vi "Append Image to Report (path).vi"(0 "report in":refnum<class "ooWriter.lvclass">, 1 "alignment (default)":T1, 2 "MS Office parameters":T2, 7 "path or URL of image":path, 9 "caption or alternative string":string, 11 "error in (no error)":errorcluster) -> (4 "report out":refnum<class "ooWriter.lvclass">, 8 "start out (Word)":i32, 10 "end out (Word)":i32, 15 "error out":errorcluster)   [LabVIEW 2009, in "ooWriter.lvclass"]
doc: "For an HTML report, the VI embeds a link to an image into the report. For a standard report, the VI appends the image from a file. You can wire either a path to the image or a string that contains the image URL to this polymorphic VI. The data type you wire to the <B>path or URL of image</B> input determines the polymorphic instance to use."
uses:
  ooWriter.lvclass
  <vilib>/Utility/NIReport.llb/HTML Report Image Alignment.ctl
  C:/Projets/LAVAG/OpenOfficeRGT/AODL/DLLs/AODL.dll
  ooWriter.lvclass/ooWriter.ctl
  <vilib>/Utility/NIReport.llb/NI_ReportGenerationCore.lvlib
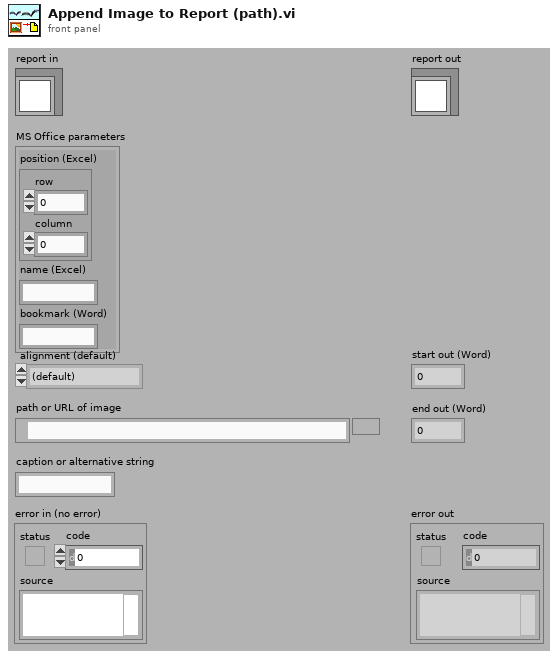
[diagram p1: front panel]
types:
  T1 = typedef "NI_ReportGenerationCore.lvlib/HTML Report Image Alignment.ctl" = enum16{"(default)", "LEFT", "RIGHT", "TOP", "TEXTTOP", "MIDDLE", "ABSMIDDLE", "BASELINE", "BOTTOM", "ABSBOTTOM"}
  T2 = cluster{"position (Excel)":cluster{"row":i32, "column":i32}, "name (Excel)":string, "bookmark (Word)":string}
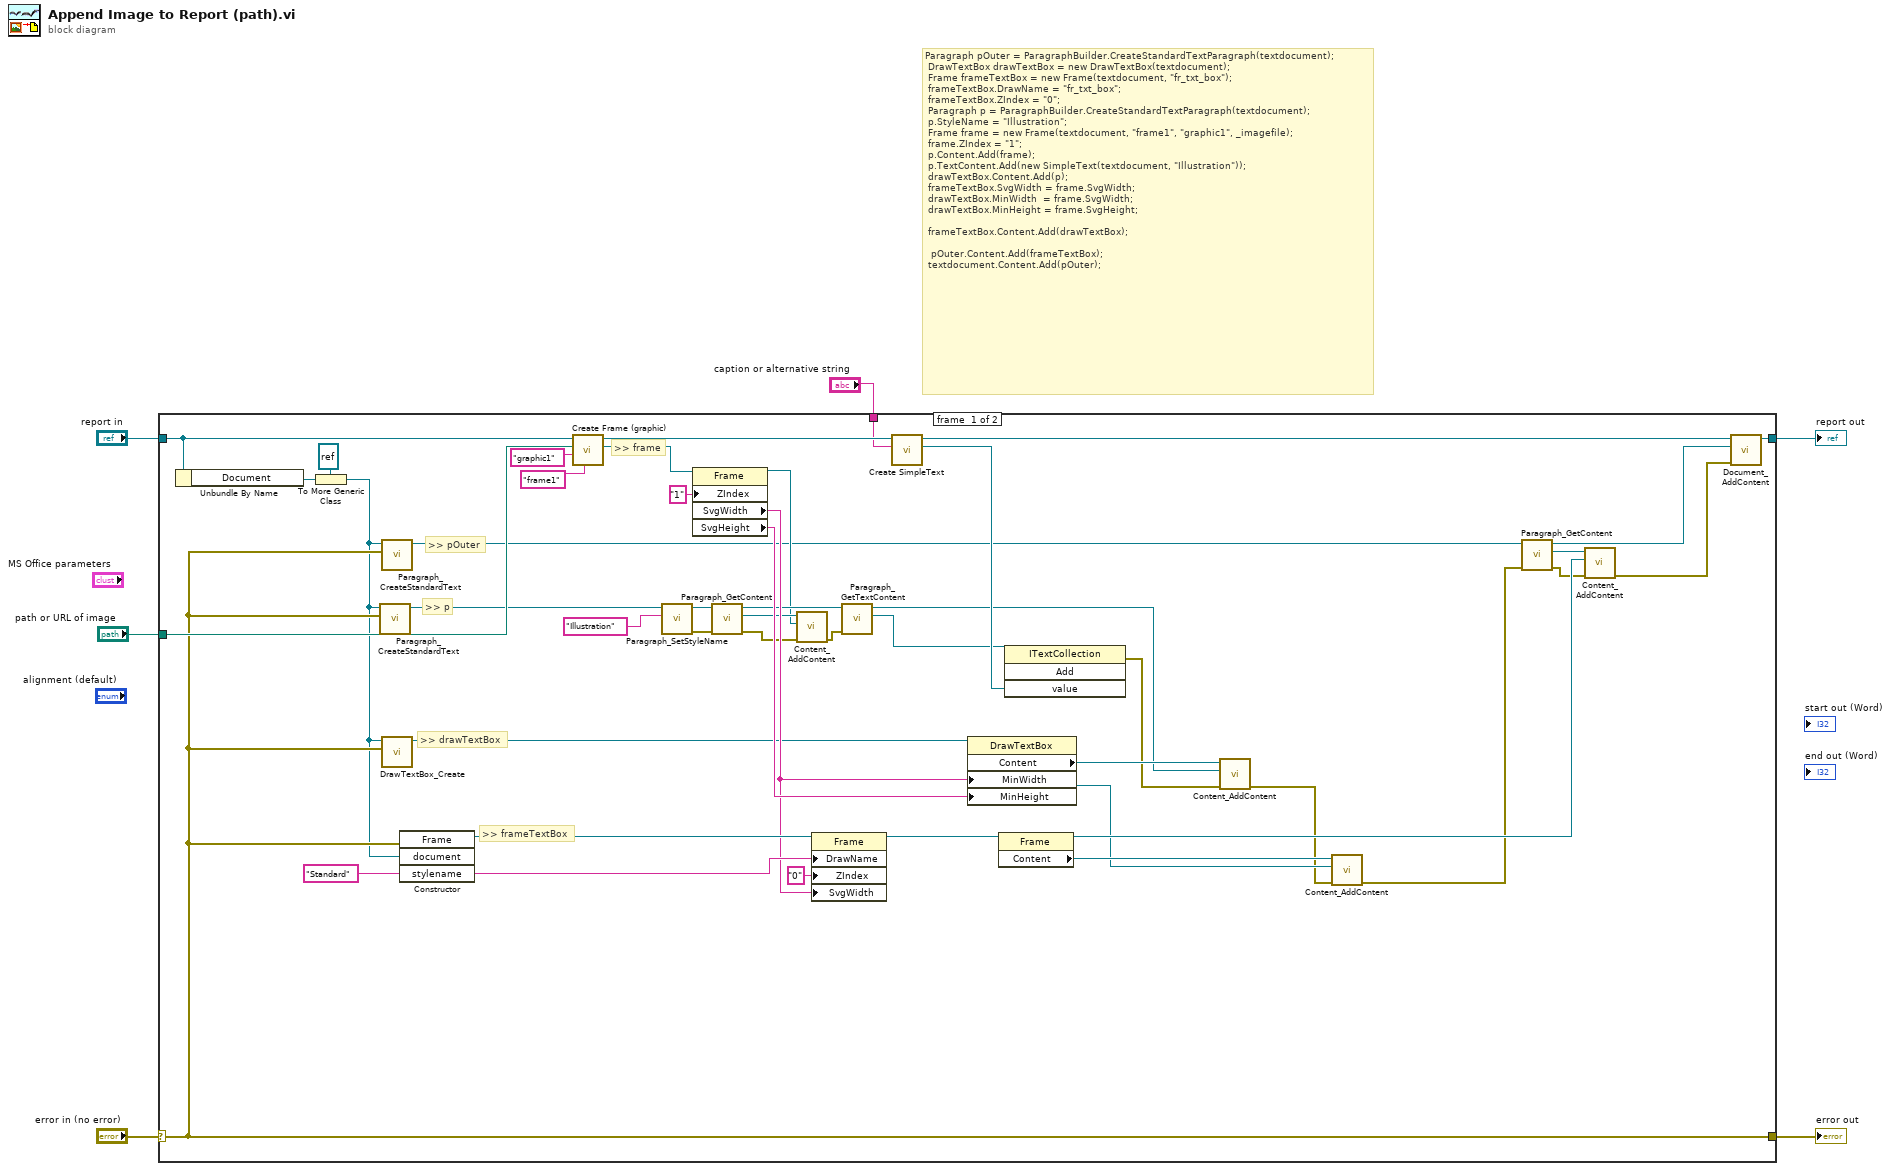
[diagram p0: block diagram]
diagram:
  # "Paragraph pOuter = ParagraphBuilder.CreateStandardTextParagraph(textdocument);\n DrawTextBox drawTextBox = new DrawTextBox(textdocument);\n Frame frameTextBox = new Frame(textdocument, \"fr_txt_box\");\n frameTextBox.DrawName = \"fr_txt_box\";\n frameTextBox.ZIndex = \"0\";\n Paragraph p = ParagraphBuilder.CreateStandardTextParagraph(textdocument);\n p.StyleName = \"Illustration\";\n Frame frame = new Frame(textdocument, \"frame1\", \"graphic1\", _imagefile);\n frame.ZIndex = \"1\";\n p.Content.Add(frame);\n p.TextContent.Add(new SimpleText(textdocument, \"Illustration\"));\n drawTextBox.Content.Add(p);\n frameTextBox.SvgWidth = frame.SvgWidth;\n drawTextBox.MinWidth  = frame.SvgWidth;\n drawTextBox.MinHeight = frame.SvgHeight;\n\n frameTextBox.Content.Add(drawTextBox);\n\n  pOuter.Content.Add(frameTextBox);\n textdocument.Content.Add(pOuter);"
  n1 = case shown="No Error" "error in (no error)" {
    selector: "error in (no error)" -> [w11 w52]
    tunnel: [w11 w52] -> w5
    tunnel: "report in" -> [w17 w53]
    tunnel: [w51 w53] -> w3
    tunnel: "path or URL of image" -> [w46 _]
    tunnel: "caption or alternative string" -> [w36 _]
    frame #0 {
      w49 = "Standard" ("frameStyleName")
      # ">> frame"
      # ">> p"
      # ">> frameTextBox"
      # ">> drawTextBox"
      # ">> pOuter"
      n2 = Unbundle By Name(w17) -> ("Document"=w8:refnum<k24>)
      n3 = To More Generic Class(target class=refnum<k24> refnum, reference=w8) -> (generic class reference=w7:refnum<k24>)
      n4 = call "Paragraph_CreateStandardText.vi"("error in"=w11, "document"=w7) -> ("StandardTextParagraph"=w18:refnum<k24>)  [unwired: 8 in, 1 out]
      n5 = call "Paragraph_CreateStandardText.vi"("error in"=w11, "document"=w7) -> ("StandardTextParagraph"=w16:refnum<k24>)  [unwired: 8 in, 1 out]
      n6 = call "DrawTextBox_Create.vi"("error in"=w11, "document"=w7) -> ("DrawTextBox"=w10:refnum<k24>)  [unwired: 8 in, 1 out]
      n7 = constructor class="Frame"(error in=w11, "document"=w7, "stylename"=w49) -> (reference out=w50:refnum<k24>)  [unwired: 2 in, 4 out]
      n8 = call-dynamic "Create Frame (graphic).vi"("stylename"="frame1", "drawName"="graphic1", "Graphic file"=w46, "ooWriter in"=w17) -> ("Frame (graphic)"=w42:refnum<k24>, "ooWriter out"=w39:refnum<class "ooWriter.lvclass">)  [unwired: 5 in, 1 out]
      n9 = call "Paragraph_SetStyleName.vi"("StyleName"="Illustration", "Paragraph"=w18) -> ("error out"=w29:errorcluster, "Paragraph dup"=w33:refnum<k24>)  [unwired: 8 in]
      n10 = property class="Frame"(reference=w42, "ZIndex"="1") -> (reference out=w30:refnum<k24>, "SvgWidth"=w40:string, "SvgHeight"=w41:string)  [unwired: 1 in, 1 out]
      n11 = call "Paragraph_GetContent.vi"("error in"=w29, "Paragraph"=w33) -> ("error out"=w27:errorcluster, "ContentCollection"=w31:refnum<k24>, "Paragraph dup"=w35:refnum<k24>)  [unwired: 7 in]
      n12 = call "Content_AddContent.vi"("error in"=w27, "Content"=w30, "ContentCollection"=w31) -> ("error out"=w28:errorcluster)  [unwired: 7 in, 1 out]
      n13 = property class="Frame"(reference=w50, "DrawName"=w49, "ZIndex"="0", "SvgWidth"=w40) -> (reference out=w47:refnum<k24>)  [unwired: 1 in, 1 out]
      n14 = call "Paragraph_GetTextContent.vi"("error in"=w28, "Paragraph"=w35) -> ("TextContent Collection"=w34:refnum<k24>, "Paragraph dup"=w22:refnum<k24>)  [unwired: 7 in, 1 out]
      n15 = call-dynamic "Create SimpleText.vi"("simpleText"=w36, "ooWriter in"=w39) -> ("SimpleText"=w37:refnum<k24>, "ooWriter out"=w38:refnum<class "ooWriter.lvclass">)  [unwired: 7 in, 1 out]
      n16 = property class="DrawTextBox"(reference=w10, "MinWidth"=w40, "MinHeight"=w41) -> (reference out=w20:refnum<k24>, "Content"=w24:refnum<k24>)  [unwired: 1 in, 1 out]
      n17 = property class="Frame"(reference=w47) -> (reference out=w26:refnum<k24>, "Content"=w21:refnum<k24>)  [unwired: 1 in, 1 out]
      n18 = invoke class="ITextCollection" method="Add"(reference=w34, "value"=w37) -> (error out=w23:errorcluster)  [unwired: 2 in, 3 out]
      n19 = call "Content_AddContent.vi"("error in"=w23, "Content"=w22, "ContentCollection"=w24) -> ("error out"=w19:errorcluster)  [unwired: 7 in, 1 out]
      n20 = call "Content_AddContent.vi"("error in"=w19, "Content"=w20, "ContentCollection"=w21) -> ("error out"=w12:errorcluster)  [unwired: 7 in, 1 out]
      n21 = call "Paragraph_GetContent.vi"("error in"=w12, "Paragraph"=w16) -> ("error out"=w13:errorcluster, "ContentCollection"=w14:refnum<k24>, "Paragraph dup"=w15:refnum<k24>)  [unwired: 7 in]
      n22 = call "Content_AddContent.vi"("error in"=w13, "Content"=w26, "ContentCollection"=w14) -> ("error out"=w25:errorcluster)  [unwired: 7 in, 1 out]
      n23 = call-dynamic "Document_AddContent.vi"("error in (no error)"=w25, "Content"=w15, "ooWriter in"=w38) -> ("ooWriter out"=w51:refnum<class "ooWriter.lvclass">)  [unwired: 7 in, 1 out]
    }
    frame #1 {
    }
  }
  "error out" <- w5
  "report out" <- w3
